vi "ConnectCore.vi"(8 "error in (no error)":errorcluster, 10 "Connection String":string, 11 "GRPCClient in":refnum<class "MicronGRPCClient.lvclass">) -> (0 "error out":errorcluster, 3 "GRPCClient out":refnum<class "MicronGRPCClient.lvclass">)   [LabVIEW 2019, in "MicronGRPCClient.lvclass"]
uses:
  MicronGRPCClient.lvclass
  MicronGRPCClient.lvclass/MicronGRPCClient.ctl
  Generated/MicronGRPCGeneratedClient/MicronGRPCGeneratedClient.lvlib
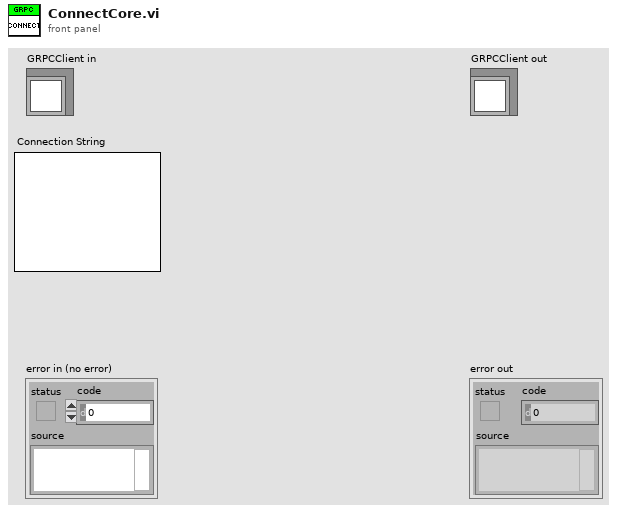
[diagram p1: front panel]
types:
  T1 = typedef "grpc-lvsupport-release.lvlib/grpcId.ctl" = u64
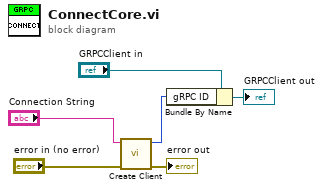
[diagram p0: block diagram]
diagram:
  n1 = call "Create Client.vi"("error in"="error in (no error)", "address"="Connection String") -> ("error out"=→"error out":errorcluster, "gRPC ID Out"=w3:T1)  [unwired: 8 in]
  n2 = Bundle By Name(cluster="GRPCClient in", "gRPC ID"=w3) -> (→"GRPCClient out":refnum<class "MicronGRPCClient.lvclass">)
